vi "Configure Signaling TDD Periodicity.vi"(7 "Periodicity (0.5 ms)":i32(ring) items=["0.5 ms", "1 ms", "1.25 ms", "2 ms", "2.5 ms", "3 ms", "4 ms", "5 ms", "10 ms"], 8 "error in (no error)":errorcluster, 9 "Pattern (1)":T1=1, 10 "Cell Name (\"Cell Name\")":string="Cell Name", 11 "VISA resource name":refnum<visa-resource-name>) -> (0 "error out":errorcluster, 3 "VISA resource name out":refnum<visa-resource-name>)   [LabVIEW 2020, in "Rohde&Schwarz CMWXP NR FR1 Measurement.lvlib"]
doc: "Configures the periodicity of the UL-DL pattern <p>.\n\nAttribute:\nRSCMWXPNRFR1M_ATTR_SIGNALING_TDD_PERIODICITY\n\nRemote-control command:\n[CONFigure:]SIGNaling:NRADio:CELL:TDD:PATTern<p>:PERiodicity"
uses:
  <instrlib>/Rohde&Schwarz CMWXP NR FR1 Measurement/Rohde&Schwarz CMWXP NR FR1 Measurement.lvlib
  <instrlib>/Rohde&Schwarz CMWXP NR FR1 Measurement/Private/_Pattern.ctl
  <instrlib>/Rohde&Schwarz CMWXP NR FR1 Measurement/Private/rsidr_core.llb/rsidr_core.lvlib
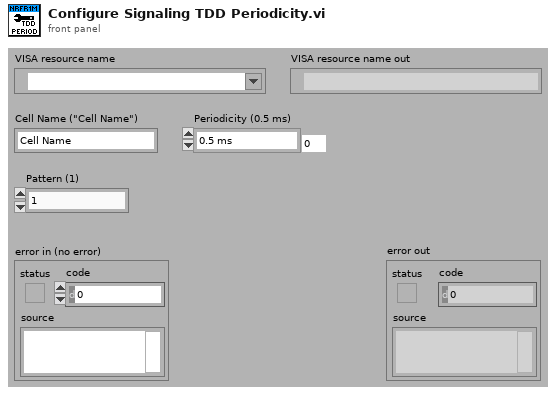
[diagram p1: front panel]
types:
  T1 = typedef "Rohde&Schwarz CMWXP NR FR1 Measurement.lvlib/_Pattern.ctl" = i32
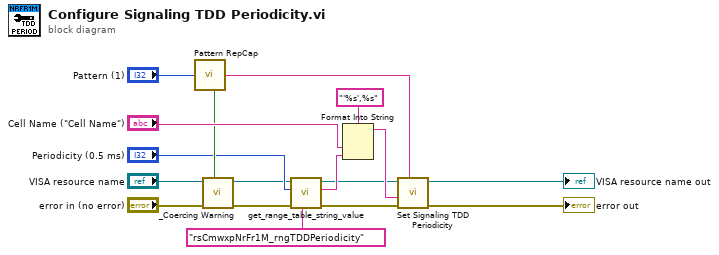
[diagram p0: block diagram]
diagram:
  n1 = call <instrlib>:"Pattern RepCap.vi"("Pattern In"="Pattern (1)") -> ("In Range?"=w8:bool, "RepCap Identifier Out"=w13:string)  [unwired: 1 in]
  n2 = call <instrlib>:"_Coercing Warning.vi"("In Range?"=w8, "error in (no error)"="error in (no error)", "VISA resource name"="VISA resource name") -> ("error out"=w5:errorcluster, "VISA resource name out"=w4:refnum<visa-resource-name>)  [unwired: 7 in]
  n3 = call <instrlib>:"get_range_table_string_value.vi"("Range Table ID in"="rsCmwxpNrFr1M_rngTDDPeriodicity", "error in"=w5, "I32 input"="Periodicity (0.5 ms)", "VISA resource name"=w4) -> ("error out"=w3:errorcluster, "String Value out"=w6:string, "VISA resource name out"=w2:refnum<visa-resource-name>)  [unwired: 5 in]
  n4 = Format Into String(format string="'%s',%s", "Cell Name (\"Cell Name\")", w6) -> (resulting string=w11:string)  [unwired: 2 in, 1 out]
  n5 = call "Set Signaling TDD Periodicity"("Repeated Capabilities"=w13, "error in (no error)"=w3, "Signaling TDD Periodicity ()"=w11, "instrument handle"=w2) -> ("error out"=→"error out":errorcluster, "instrument handle out"=→"VISA resource name out":refnum<visa-resource-name>)  [unwired: 6 in]
